vi "DLCpro example - SHG.vi"() -> ()   [LabVIEW 2013]
panel:
  out "error out":errorcluster
  in  "Tab Control 2":enum32{"Page 1"}(tab)
  in  "Port":string="1998"
  in  "IP Address of DLC pro":string="192.168.1.200"
  in  "COM port":refnum<visa-resource-name>="COM1"
  in  "Connect":bool
  in  "connection":enum32{"TCP/IP", "USB"}(radio)
  out "Serial number":string
  out "Status":string
  in  "Password":string="Your password"
  out "Graph Channel2":T1(graph)
  out "Graph Channel1":T1(graph)
  in  "Quit?":bool
  in  "Tab Control":enum32{"Amplifier Power", "SHG Power"}(tab)
  out "Progress [%]":u32(slide) scale=0.0..100.0
  in  "Start Opt Amp":bool
  out "answer string":string
  out "Waveform Graph 2":sgl[](graph)
  in  "Start Opt SHG":bool
  out "answer string":string
  out "Progress [%]":u32(slide) scale=0.0..100.0
  out "Waveform Graph":sgl[](graph)
  # "Connection"
  # "Power Graphs"
  # "WARNING!\nConnecting to a DLC pro will alter its Scope settings, by using the following parameters:\n\n-laser1:scope:channel1:enabled\n-laser1:scope:channel1:signal\n-laser1:scope:channel2:enabled\n-laser1:scope:channel2:signal\n\n-laser1:scope:channelx:xy-signal\n-laser1:scope:variant\n\n-laser1:nlo:shg:lock:lock-enabled\n-laser1:nlo:power-optimization:start-optimization-shg\n-laser1:nlo:power-optimization:start-optimization-amp\n\n1. Connecting to the DLC pro\n \na) Connection via TCP/IP\n\nWrite the IP Address of your DLC pro into the input field \"IP Address\" (e.g., 192.168.1.200).\n \nNOTE!\nThe DLC pro has to be connected to a local area network (LAN) or directly to a PC \n(e.g., with a cross link cable).  Further, the DLC pro and the PC must have the same \nsubnet mask and different IP addresses. You can edit these parameters of your\ndevice in the section \"Network Settings\" on your DLC pro. To connect the DLC pro \ndirectly to a computer, disable DHCP on both devices, set the same subnet mask \n(e.g., 255.255.255.0) and different IP addresses (e.g., 192.168.1.200 and 192.168.1.201)\n\n\nb) Connection via USB\n\nSelect the virtual COM port of your DLC pro in the field \"COM port\" (e.g., COM1).\n\nNOTE!\nFor DLC pro control via USB, the control computer must be connected to the USB connector at the MC/MC+ module via a micro USB cable with connector type B. Further, a specific USB driver has to be installed on your computer. When connecting your DLC pro to a USB port of your PC, it will be identified as a \"DLCpro\" device  and registered as a virtual COM port.\nDriver insatllation:\n- Make sure that the DLC pro is not connected with the control computer via  USB.  \n- You need two files for the installation of the driver which you find on your TOPTICA USB stick in the folder \"2_PC_GUI_...\". Their names are \"dlcpro-usb-serial.cat\" and \"dlcpro-usb-serial.inf\".\n- To install the driver, copy both files to the same location on your computer, right-click \n\"dlcpro-usb-serial.inf\", click \"install\", and confirm the installation in the dialog window.\n\n\n2. Start the program. If you can see the serial number of your DLC pro the connection was successful. If you have assigned a password for your device insert it to the field \"Password\". If you didn't assign a password you can ignore this field. The \"Status\" indicator should show \"READY\" now.\n\n\n3. The graph shows an example how to retrieve data traces from the DLC pro device, in this case the \"SHG Power \" and \"Amplifier Power \" traces. \n\n4. Start the  Power Optimization for the Amplifier or the SHG by clicking on the Start button In the tab-window. You can watch the progress by the bar or the Optimization Iteration Graph. The answer string returns the answer of the execute command. Usually it is \"0\".\n\n5. Stop the program and close the existing connection by pushing the \"STOP & CLOSE CONNECTION\" button."
  # "Power Optimization"
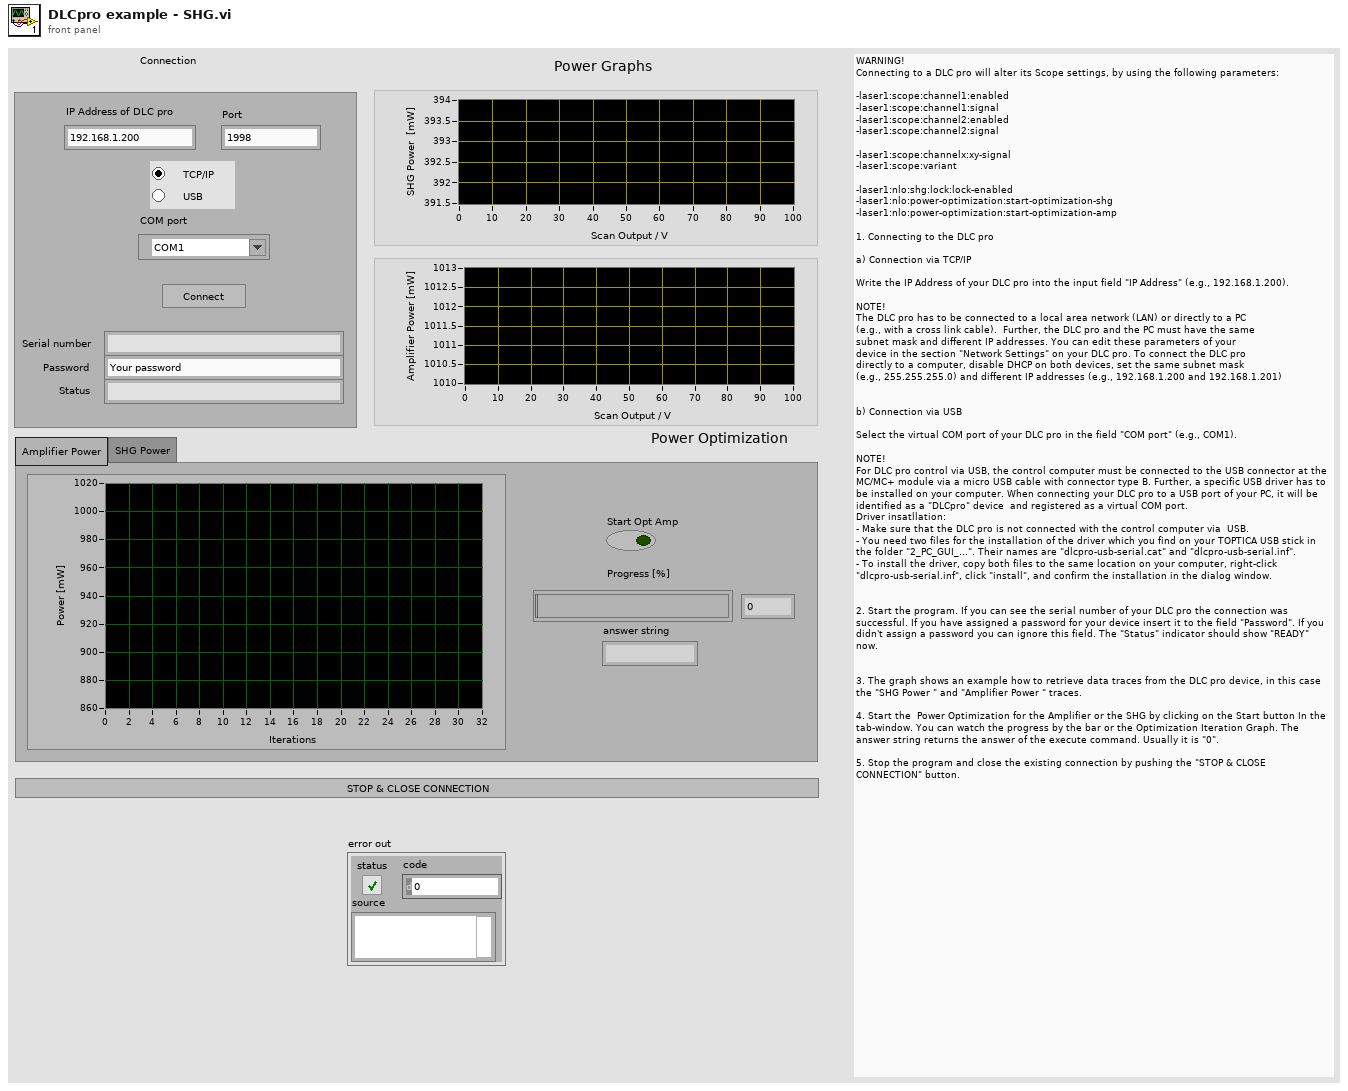
[diagram p1: front panel]
types:
  T1 = cluster{"Channel 1 data":sgl[], "Channel2 data":sgl[]}
  T2 = enum8{"Enabled", "Disabled", "Disabled and Grayed Out"}
  T3 = typedef "DeCoF connection.ctl" = cluster{"TCP/IP":bool, "VISA":refnum<visa-resource-name>, "TCP/IP ID":refnum<k5>}
  T4 = enum16{"big-endian, network order", "native, host order", "little-endian"}
  T5 = cluster{"float array":sgl[], "float array":sgl[]}
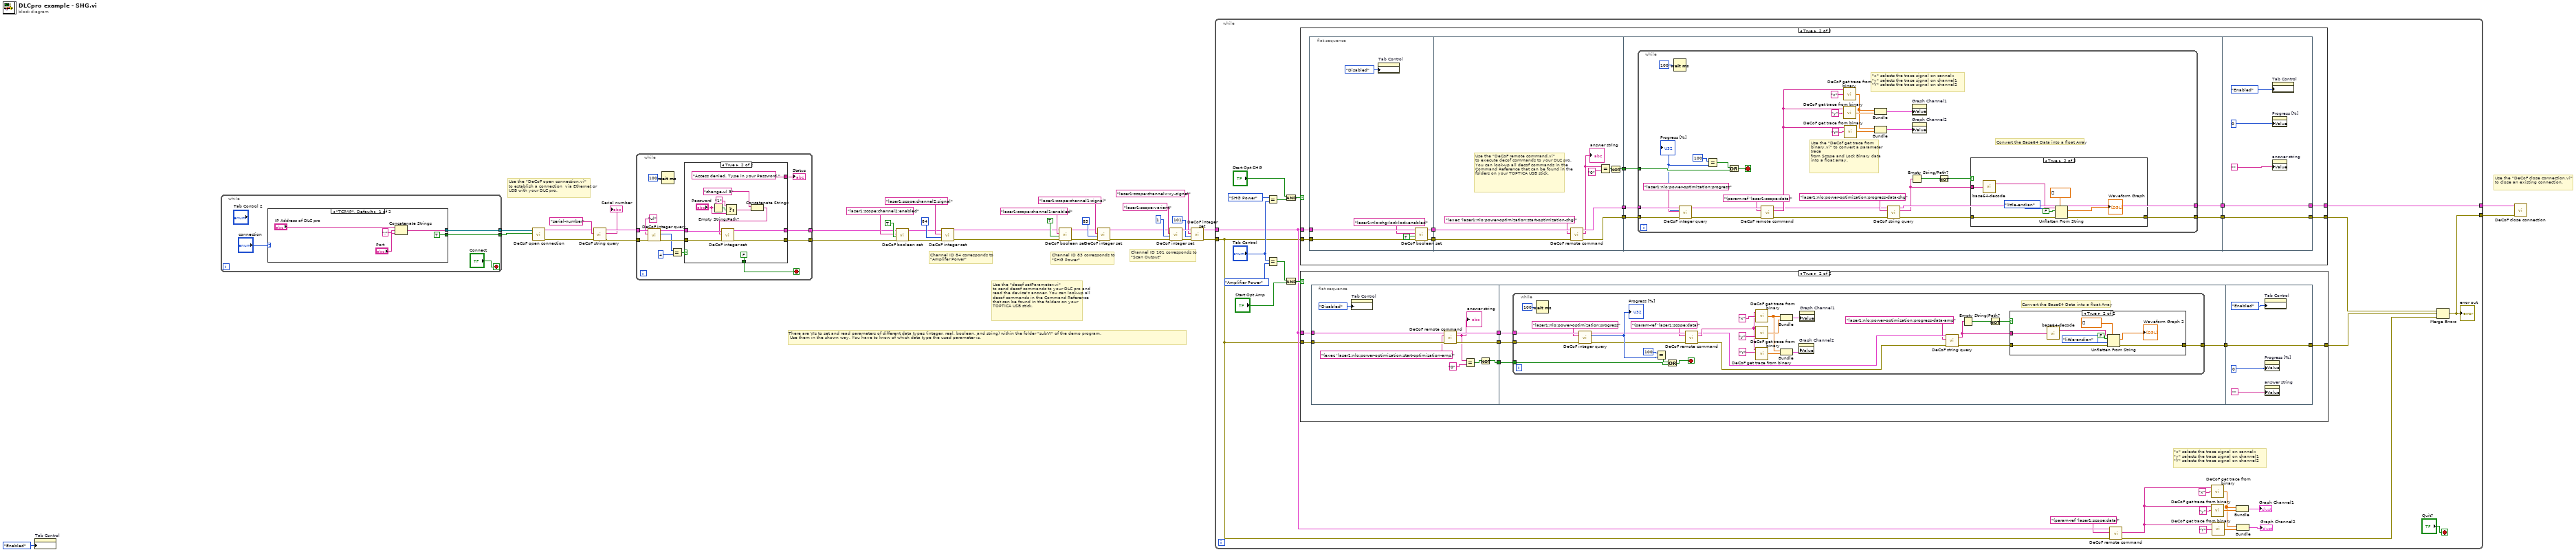
[diagram p0: block diagram]
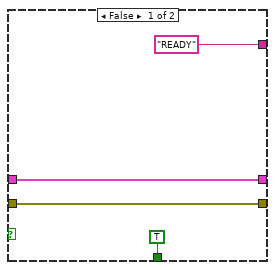
[diagram p2: hidden frame]
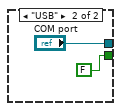
[diagram p3: hidden frame]
diagram:
  # "Channel ID 101 corresponds to\n\"Scan Output\""
  # "Use the \"DeCoF close connection.vi\"\nto close an existing connection."
  # "Channel ID 83 corresponds to\n\"SHG Power\""
  # "Channel ID 84 corresponds to\n\"Amplifer Power\""
  # "There are VIs to set and read parameters of different data types (integer, real, boolean, and string) within the folder \"subVI\" of the demo program. \n Use them in the shown way. You have to know of which data type the used parameter is."
  # "Use the \"decof setParameter.vi\"\nto send decof commands to your DLC pro and read the device's answer. You can look-up all decof commands in the Command Reference that can be found in the folders on your TOPTICA USB stick."
  # "Use the \"DeCoF open connection.vi\"\nto establish a connection  via Ethernet or USB with your DLC pro."
  n1 = property on="Tab Control" class="TabCtl (strict)"("DisabledEnum"=T2."Enabled" ("Disabled")) -> ()  [unwired: 2 in, 2 out]
  n2 = while {
    tunnel: [w40] -> w35
    tunnel: [w39] -> w36
    stop <- "Connect" stop-if-true
    n3 = case shown="\"TCP/IP\", Default" "connection" {
      tunnel: [w42 "COM port"] -> w39
      tunnel: [TRUE FALSE] -> w40
      frame "TCP/IP", Default {
        n4 = Concatenate Strings("IP Address of DLC pro", ":" ("string"), "Port") -> (w42:string)
      }
      frame "USB" {
      }
    }
  }
  n5 = call "DeCoF open connection.vi"("TCP?"=w35, "address"=w36) -> ("error out"=w8:errorcluster, "Conncection ID out"=w6:T3)  [unwired: 4 in]
  n6 = call "DeCoF string query.vi"("error in"=w8, "param-name"="serial-number" ("command"), "Conncection ID in"=w6) -> ("error out"=w9:errorcluster, "value"=→"Serial number":string, "Conncection ID out"=w5:T3)  [unwired: 2 in]
  n7 = while {
    tunnel: w5 -> [w52]
    tunnel: w9 -> [w53]
    tunnel: [w57] -> w10
    tunnel: [w56] -> w13
    stop <- w59 stop-if-true
    n8 = call "DeCoF integer query.vi"("error in"=w53, "param-name"="ul", "Conncection ID in"=w52) -> ("error out"=w50:errorcluster, "value"=w49:i32, "Conncection ID out"=w54:T3)  [unwired: 2 in]
    n9 = Wait (ms)(milliseconds to wait=u32 100) -> ()  [unwired: 1 out]
    n10 = Equal?(x=w49, y=4) -> (x = y?=w61:bool)
    n11 = case shown="True" w61 {
      tunnel: [TRUE FALSE] -> w59
      tunnel: w54 -> [w64 w68]
      tunnel: [w64 w66] -> w57
      tunnel: w50 -> [w63 w69]
      tunnel: [w63 w70] -> w56
      tunnel: ["READY" "Access denied. Type in your Password."] -> w58
      frame False {
      }
      frame True {
        n12 = Empty String/Path?(string/path="Password") -> (empty?=w74:bool)
        n13 = Select(t="1", s=w74, f="Password") -> (s? t:f=w71:string)
        n14 = Concatenate Strings("change-ul 3", w71) -> (w67:string)
        n15 = call "DeCoF integer set.vi"("error in"=w69, "param-name"=w67, "Conncection ID in"=w68) -> ("error out"=w70:errorcluster, "Conncection ID out"=w66:T3)  [unwired: 3 in]
      }
    }
    "Status" <- w58
  }
  n16 = call "DeCoF boolean set.vi"("error in"=w13, "value"=TRUE ("input value"), "param-name"="laser1:scope:channel2:enabled", "Conncection ID in"=w10) -> ("error out"=w14:errorcluster, "Conncection ID out"=w15:T3)  [unwired: 2 in]
  n17 = call "DeCoF integer set.vi"("error in"=w14, "value"=84 ("input value"), "param-name"="laser1:scope:channel2:signal", "Conncection ID in"=w15) -> ("error out"=w21:errorcluster, "Conncection ID out"=w18:T3)  [unwired: 2 in]
  n18 = call "DeCoF boolean set.vi"("error in"=w21, "value"=TRUE ("input value"), "param-name"="laser1:scope:channel1:enabled", "Conncection ID in"=w18) -> ("error out"=w23:errorcluster, "Conncection ID out"=w22:T3)  [unwired: 2 in]
  n19 = call "DeCoF integer set.vi"("error in"=w23, "value"=83 ("input value"), "param-name"="laser1:scope:channel1:signal", "Conncection ID in"=w22) -> ("error out"=w26:errorcluster, "Conncection ID out"=w27:T3)  [unwired: 2 in]
  n20 = call "DeCoF integer set.vi"("error in"=w26, "value"=1 ("input value"), "param-name"="laser1:scope:variant", "Conncection ID in"=w27) -> ("error out"=w32:errorcluster, "Conncection ID out"=w33:T3)  [unwired: 2 in]
  n21 = call "DeCoF integer set.vi"("error in"=w32, "value"=101 ("input value"), "param-name"="laser1:scope:channelx:xy-signal" ("parameter name"), "Conncection ID in"=w33) -> ("error out"=w1:errorcluster, "Conncection ID out"=w34:T3)  [unwired: 2 in]
  n22 = while {
    tunnel: w34 -> [w79]
    tunnel: [w90] -> w2
    tunnel: [w89] -> w3
    tunnel: w1 -> [w78]
    stop <- "Quit?" stop-if-true
    # "\"x\" selects the trace signal on cannelx\n\"y\" selects the trace signal on channel1\n\"Y\" selects the trace signal on channel2"
    n23 = Equal?(x=enum32{"Amplifier Power", "SHG Power"}."SHG Power", y="Tab Control") -> (x = y?=w86:bool)
    n24 = Equal?(x="Tab Control", y=enum32{"Amplifier Power", "SHG Power"}."Amplifier Power") -> (x = y?=w103:bool)
    n25 = And(x="Start Opt SHG", y=w86) -> (x .and. y?=w100:bool)
    n26 = And(x=w103, y="Start Opt Amp") -> (x .and. y?=w101:bool)
    n27 = case shown="True" w100 {
      tunnel: w79 -> [w105 w117]
      tunnel: w78 -> [w106 w115]
      tunnel: [w106 w112] -> w99
      tunnel: [w105 w109] -> w90
      frame False {
      }
      frame True {
        n28 = flat-sequence {
          tunnel: w115 -> [w120]
          tunnel: w117 -> [w123]
          tunnel: [w118] -> w111
          tunnel: [w119] -> w110
          tunnel: [w129] -> w116
          tunnel: [w128] -> w114
          tunnel: w111 -> [w130]
          tunnel: w110 -> [w127]
          tunnel: [w131] -> w107
          tunnel: w116 -> [w138]
          tunnel: w114 -> [w137]
          tunnel: [w136] -> w113
          tunnel: [w135] -> w108
          tunnel: w107 -> [w134]
          tunnel: [w180] -> w112
          tunnel: w113 -> [w180]
          tunnel: [w179] -> w109
          tunnel: w108 -> [w179]
          frame #0 {
            n29 = property on="Tab Control" class="TabCtl (strict)"("DisabledEnum"=T2."Disabled" ("Disabled")) -> ()  [unwired: 2 in, 2 out]
            n30 = call "DeCoF boolean set.vi"("error in"=w120, "value"=TRUE ("input value"), "param-name"="laser1:nlo:shg:lock:lock-enabled" ("parameter name"), "Conncection ID in"=w123) -> ("error out"=w119:errorcluster, "Conncection ID out"=w118:T3)  [unwired: 2 in]
          }
          frame #1 {
            # "Use the \"DeCoF remote command.vi\"\nto execute decof commands to your DLC pro. You can look-up all decof commands in the Command Reference that can be found in the folders on your TOPTICA USB stick."
            n31 = call "DeCoF remote command.vi"("error in (no error)"=w127, "command"="(exec 'laser1:nlo:power-optimization:start-optimization-shg)" ("command parameter string"), "Conncection ID in"=w130) -> ("error out"=w128:errorcluster, "answer string"=w126:string, "Conncection ID out"=w129:T3)  [unwired: 2 in, 2 out]
            "answer string" <- w126
            n32 = Equal?(x=w126, y="0") -> (x = y?=w132:bool)
            n33 = Not(x=w132) -> (.not. x?=w131:bool)
          }
          frame #2 {
            n34 = while {
              tunnel: w138 -> [w154]
              tunnel: w137 -> [w153]
              tunnel: [w142] -> w136
              tunnel: [w143] -> w135
              tunnel: w134 -> [w157]
              stop <- w156 stop-if-true
              # "Use the \"DeCof get trace from binary.vi\" to convert a parameter trace \nfrom Scope and Lock Binary data  into a float array."
              # "Convert the Base64 Data into a float Array"
              # "\"x\" selects the trace signal on cannelx\n\"y\" selects the trace signal on channel1\n\"Y\" selects the trace signal on channel2"
              n35 = Wait (ms)(milliseconds to wait=u32 100) -> ()  [unwired: 1 out]
              n36 = call "DeCoF integer query.vi"("error in"=w153, "param-name"="laser1:nlo:power-optimization:progress" ("parameter name"), "Conncection ID in"=w154) -> ("error out"=w149:errorcluster, "value"=w151:i32, "Conncection ID out"=w150:T3)  [unwired: 2 in]
              "Progress [%]" <- w151
              n37 = Equal?(x=100, y=w151) -> (x = y?=w158:bool)
              n38 = Or(x=w158, y=w157) -> (x .or. y?=w156:bool)
              n39 = call "DeCoF remote command.vi"("error in (no error)"=w149, "command"="(param-ref 'laser1:scope:data)" ("parameter name"), "Conncection ID in"=w150) -> ("error out"=w146:errorcluster, "answer string"=w148:string, "Conncection ID out"=w144:T3)  [unwired: 2 in, 2 out]
              n40 = call "DeCoF get trace from binary.vi"("Block ID"="x" ("identifier 1"), "Binary in"=w148) -> ("float array"=w162:sgl[])  [unwired: 1 in]
              n41 = call "DeCoF get trace from binary.vi"("Block ID"="y", "Binary in"=w148) -> ("float array"=w164:sgl[])  [unwired: 1 in]
              n42 = call "DeCoF get trace from binary.vi"("Block ID"="Y", "Binary in"=w148) -> ("float array"=w155:sgl[])  [unwired: 1 in]
              n43 = Bundle("float array"=w162, "float array"=w164) -> (w161:T5)  [unwired: 1 in]
              n44 = Bundle("float array"=w162, "float array"=w155) -> (w160:T5)  [unwired: 1 in]
              n45 = call "DeCoF string query.vi"("error in"=w146, "param-name"="laser1:nlo:power-optimization:progress-data-shg" ("parameter name"), "Conncection ID in"=w144) -> ("error out"=w141:errorcluster, "value"=w139:string, "Conncection ID out"=w143:T3)  [unwired: 2 in]
              n46 = Empty String/Path?(string/path=w139) -> (empty?=w159:bool)
              n47 = property on="Graph Channel1" class="XYGraph (strict)"("Value"=w161) -> ()  [unwired: 2 in, 2 out]
              n48 = property on="Graph Channel2" class="XYGraph (strict)"("Value"=w160) -> ()  [unwired: 2 in, 2 out]
              n49 = Not(x=w159) -> (.not. x?=w140:bool)
              n50 = case shown="True" w140 {
                tunnel: w139 -> [_ w177]
                tunnel: [w169 w172] -> w142
                tunnel: w141 -> [w169 w173]
                frame False {
                }
                frame True {
                  n51 = call "base64-decode.vi"("String"=w177) -> ("binary output"=w176:string)  [unwired: 1 out]
                  n52 = Unflatten From String(type=sgl[] [] ("Waveform Graph"), binary string=w176, data includes array or string size? (T)=FALSE, byte order (0:big-endian, network order)=T4."little-endian" ("byte order"), error in (no error)=w173) -> (value=→"Waveform Graph":sgl[], error out=w172:errorcluster)  [unwired: 1 out]
                }
              }
            }
          }
          frame #3 {
            n53 = property on="Tab Control" class="TabCtl (strict)"("DisabledEnum"=T2."Enabled" ("Disabled")) -> ()  [unwired: 2 in, 2 out]
            n54 = property on="Progress [%]" class="Slide (strict)"("Value"=u32 0 ("Slide 2")) -> ()  [unwired: 2 in, 2 out]
            n55 = property on="answer string" class="Str"("Value"="") -> ()  [unwired: 2 in, 2 out]
          }
        }
      }
    }
    n56 = case shown="True" w101 {
      tunnel: w79 -> [_ w190]
      tunnel: w78 -> [w183 w188]
      tunnel: [w183 w185] -> w85
      frame False {
      }
      frame True {
        n57 = flat-sequence {
          tunnel: w190 -> [w193]
          tunnel: [w194] -> w189
          tunnel: w188 -> [w196]
          tunnel: [w195] -> w187
          tunnel: [w198] -> w184
          tunnel: w189 -> [w204]
          tunnel: w187 -> [w203]
          tunnel: [w202] -> w186
          tunnel: w184 -> [w201]
          tunnel: [w244] -> w185
          tunnel: w186 -> [w244]
          frame #0 {
            n58 = property on="Tab Control" class="TabCtl (strict)"("DisabledEnum"=T2."Disabled" ("Disabled")) -> ()  [unwired: 2 in, 2 out]
            n59 = call "DeCoF remote command.vi"("error in (no error)"=w196, "command"="(exec 'laser1:nlo:power-optimization:start-optimization-amp)" ("command parameter string"), "Conncection ID in"=w193) -> ("error out"=w195:errorcluster, "answer string"=w191:string, "Conncection ID out"=w194:T3)  [unwired: 2 in, 2 out]
            "answer string" <- w191
            n60 = Equal?(x=w191, y="0") -> (x = y?=w197:bool)
            n61 = Not(x=w197) -> (.not. x?=w198:bool)
          }
          frame #1 {
            n62 = while {
              tunnel: w204 -> [w217]
              tunnel: w203 -> [w215]
              tunnel: [w223] -> w202
              tunnel: w201 -> [w219]
              stop <- w218 stop-if-true
              # "Convert the Base64 Data into a float Array"
              n63 = Wait (ms)(milliseconds to wait=u32 100) -> ()  [unwired: 1 out]
              n64 = call "DeCoF integer query.vi"("error in"=w215, "param-name"="laser1:nlo:power-optimization:progress" ("parameter name"), "Conncection ID in"=w217) -> ("error out"=w213:errorcluster, "value"=w214:i32, "Conncection ID out"=w212:T3)  [unwired: 2 in]
              "Progress [%]" <- w214
              n65 = Equal?(x=100, y=w214) -> (x = y?=w220:bool)
              n66 = Or(x=w220, y=w219) -> (x .or. y?=w218:bool)
              n67 = call "DeCoF remote command.vi"("error in (no error)"=w213, "command"="(param-ref 'laser1:scope:data)" ("parameter name"), "Conncection ID in"=w212) -> ("error out"=w208:errorcluster, "answer string"=w210:string, "Conncection ID out"=w209:T3)  [unwired: 2 in, 2 out]
              n68 = call "DeCoF get trace from binary.vi"("Block ID"="x" ("identifier 1"), "Binary in"=w210) -> ("float array"=w226:sgl[])  [unwired: 1 in]
              n69 = call "DeCoF get trace from binary.vi"("Block ID"="y", "Binary in"=w210) -> ("float array"=w229:sgl[])  [unwired: 1 in]
              n70 = call "DeCoF get trace from binary.vi"("Block ID"="Y", "Binary in"=w210) -> ("float array"=w227:sgl[])  [unwired: 1 in]
              n71 = Bundle("float array"=w226, "float array"=w229) -> (w225:T5)  [unwired: 1 in]
              n72 = Bundle("float array"=w226, "float array"=w227) -> (w224:T5)  [unwired: 1 in]
              n73 = property on="Graph Channel2" class="XYGraph (strict)"("Value"=w224) -> ()  [unwired: 2 in, 2 out]
              n74 = property on="Graph Channel1" class="XYGraph (strict)"("Value"=w225) -> ()  [unwired: 2 in, 2 out]
              n75 = call "DeCoF string query.vi"("error in"=w208, "param-name"="laser1:nlo:power-optimization:progress-data-amp" ("parameter name"), "Conncection ID in"=w209) -> ("error out"=w206:errorcluster, "value"=w205:string)  [unwired: 2 in, 1 out]
              n76 = Empty String/Path?(string/path=w205) -> (empty?=w222:bool)
              n77 = Not(x=w222) -> (.not. x?=w221:bool)
              n78 = case shown="True" w221 {
                tunnel: w205 -> [_ w242]
                tunnel: [w234 w237] -> w223
                tunnel: w206 -> [w234 w238]
                frame False {
                }
                frame True {
                  n79 = call "base64-decode.vi"("String"=w242) -> ("binary output"=w235:string)  [unwired: 1 out]
                  n80 = Unflatten From String(type=sgl[] [] ("Waveform Graph"), binary string=w235, data includes array or string size? (T)=FALSE, byte order (0:big-endian, network order)=T4."little-endian" ("byte order"), error in (no error)=w238) -> (value=→"Waveform Graph 2":sgl[], error out=w237:errorcluster)  [unwired: 1 out]
                }
              }
            }
          }
          frame #2 {
            n81 = property on="Tab Control" class="TabCtl (strict)"("DisabledEnum"=T2."Enabled" ("Disabled")) -> ()  [unwired: 2 in, 2 out]
            n82 = property on="Progress [%]" class="Slide (strict)"("Value"=u8 0 ("Slide")) -> ()  [unwired: 2 in, 2 out]
            n83 = property on="answer string" class="Str"("Value"="") -> ()  [unwired: 2 in, 2 out]
          }
        }
      }
    }
    n84 = call "DeCoF remote command.vi"("error in (no error)"=w78, "command"="(param-ref 'laser1:scope:data)" ("parameter name"), "Conncection ID in"=w79) -> ("error out"=w84:errorcluster, "answer string"=w83:string)  [unwired: 2 in, 3 out]
    n85 = call "DeCoF get trace from binary.vi"("Block ID"="x" ("identifier 1"), "Binary in"=w83) -> ("float array"=w91:sgl[])  [unwired: 1 in]
    n86 = call "DeCoF get trace from binary.vi"("Block ID"="y", "Binary in"=w83) -> ("float array"=w96:sgl[])  [unwired: 1 in]
    n87 = call "DeCoF get trace from binary.vi"("Block ID"="Y", "Binary in"=w83) -> ("float array"=w94:sgl[])  [unwired: 1 in]
    n88 = Bundle("float array"=w91, "float array"=w96) -> (→"Graph Channel1":T5)  [unwired: 1 in]
    n89 = Bundle("float array"=w91, "float array"=w94) -> (→"Graph Channel2":T5)  [unwired: 1 in]
    n90 = Merge Errors(w99, w85, w84) -> (w89:errorcluster)
    "error out" <- w89
  }
  n91 = call "DeCoF close connection.vi"("error in (no error)"=w3, "Connection ID in"=w2) -> ()  [unwired: 4 in, 2 out]
